vi "Handle getAll.vi"(8 "error in (no error)":errorcluster, 11 "Inst.AH2500 in":refnum<class "Inst.AH2500.lvclass">) -> (0 "error out":errorcluster, 2 "getAll":variant, 3 "Inst.AH2500 out":refnum<class "Inst.AH2500.lvclass">)   [LabVIEW 2019, in "Inst.AH2500.lvclass"]
uses:
  Inst.AH2500.lvclass
  Inst.AH2500.lvclass/Inst.AH2500.ctl
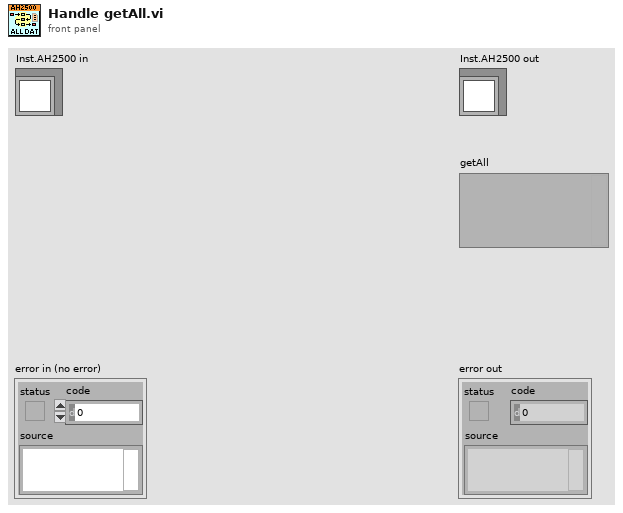
[diagram p1: front panel]
types:
  T1 = typedef "Inst.AH2500.lvclass/Inst.AH2500.getAll--Cluster.ctl" = cluster{"Output State Ch1":string, "Output State Ch2":string, "Level (V) Ch1":dbl, "Level (V) Ch2":dbl, "Slew (V/s) Ch1":dbl, "Slew (V/s) Ch2":dbl, "measured V (V) Ch1":dbl, "measured V (V) Ch2":dbl, "measured I (A) Ch1":dbl, "measured I (A) Ch2":dbl}
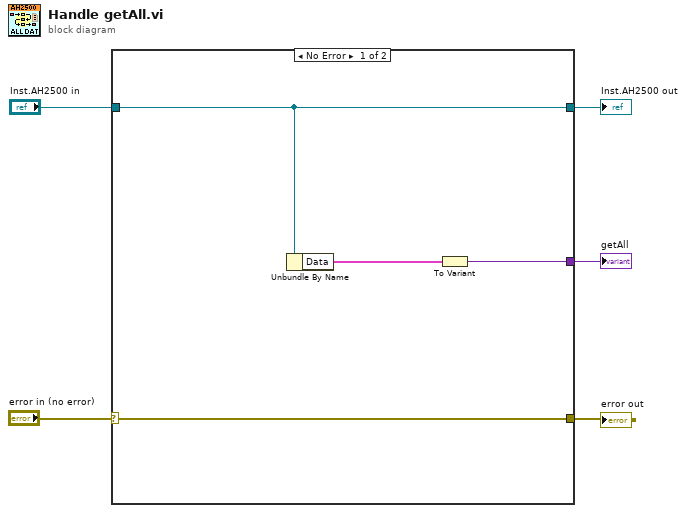
[diagram p0: block diagram]
diagram:
  n1 = case shown="No Error" "error in (no error)" {
    selector: "error in (no error)" -> [w8 w11]
    tunnel: [w8 w11] -> w3
    tunnel: [w6 w10] -> w1
    tunnel: "Inst.AH2500 in" -> [w6 w10]
    tunnel: [w9 _] -> w2
    frame No Error {
      n2 = Unbundle By Name(w6) -> ("Data"=w7:T1)
      n3 = To Variant(anything=w7) -> (Variant=w9:variant)
    }
    frame Error {
    }
  }
  "error out" <- w3
  "Inst.AH2500 out" <- w1
  "getAll" <- w2
